vi "DS345 FREQUENCY.vi"(0 "GPIB address":string="19", 1 "amplitude (0 Vrms:0)":cluster{ext, i32} {"?" items=["Vrms", "Vpp", "dBm"]; "?" format="%.3f"}, 2 "output function (sine:0)":u16(ring) items=["sine", "square", "triangle", "ramp", "noise", "arbitrary"], 3 "FREQ. units (Hz:0)":i32(ring) items=["Hz", "KHz.", "MHz."], 4 "frequency":ext format="%.6f", 5 "error in":errorcluster, 6 "phase":ext format="%.3f", 7 "DC offset":ext format="%.3f") -> (8 "error out":errorcluster)   [LabVIEW 2010]
doc: "This subVI specifies the output function, frequency , amplitude,amplitude units and phase of the DS345\nWhen the output function is set to ARBITRARY or NOISE , the frequency or phase may not be changed . \nThe frequency units are used to determine if the frequency quantity needs to be scaled up before sending it to the instrument . \nThe amplitude units can be Vpp, Vrms or dBm ."
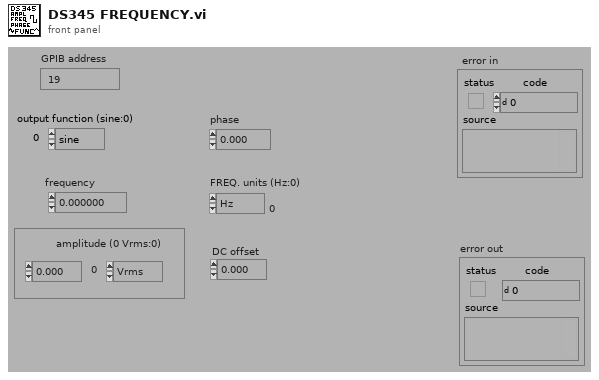
[diagram p1: front panel]
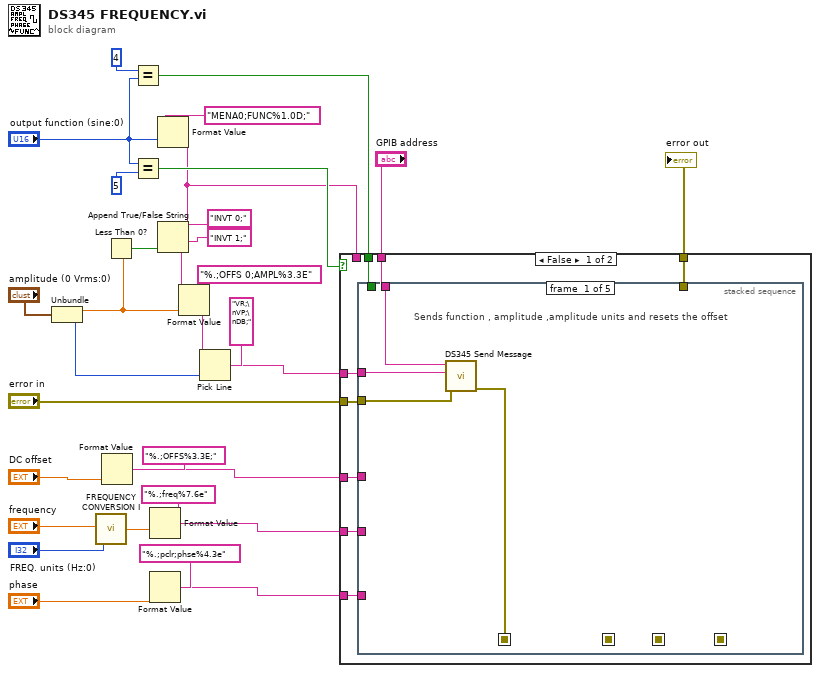
[diagram p0: block diagram]
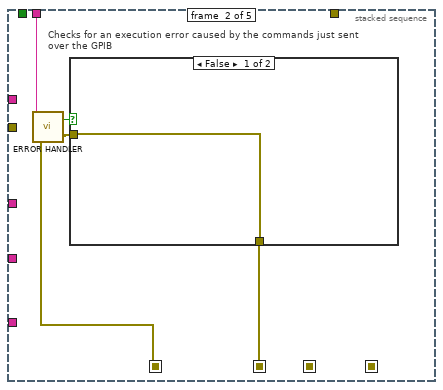
[diagram p2: hidden frame]
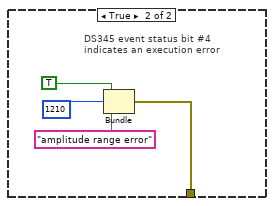
[diagram p3: hidden frame]
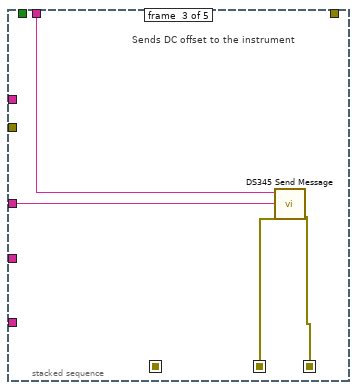
[diagram p4: hidden frame]
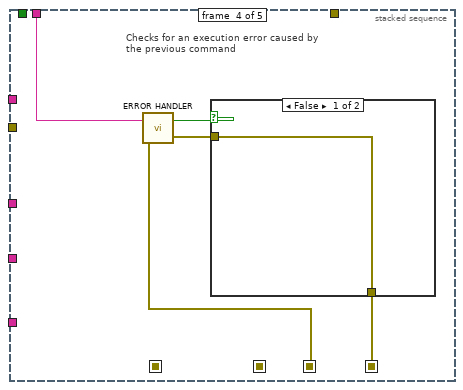
[diagram p5: hidden frame]
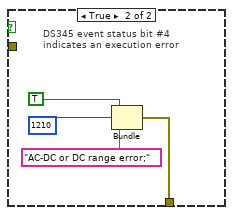
[diagram p6: hidden frame]
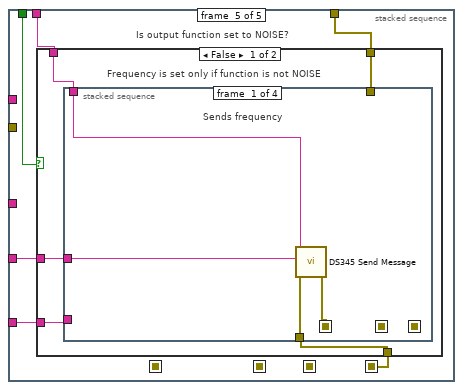
[diagram p7: hidden frame]
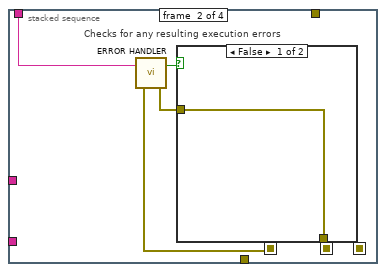
[diagram p8: hidden frame]
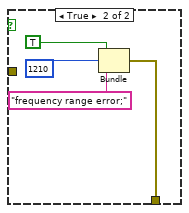
[diagram p9: hidden frame]
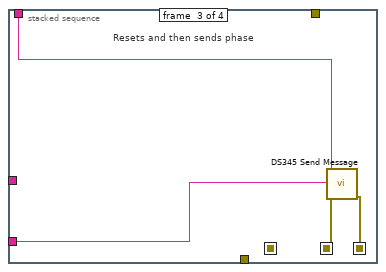
[diagram p10: hidden frame]
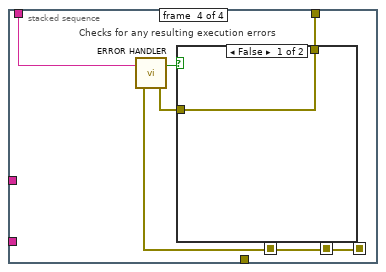
[diagram p11: hidden frame]
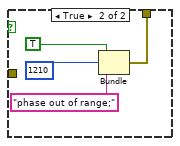
[diagram p12: hidden frame]
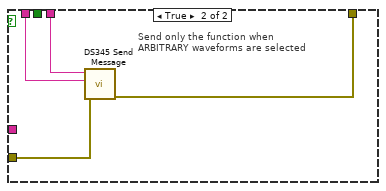
[diagram p14: hidden frame]
diagram:
  n1 = Unbundle("amplitude (0 Vrms:0)") -> (w2:ext, w22:i32)
  n2 = call "FREQUENCY CONVERSION I.vi"("unit"="FREQ. units (Hz:0)", "quantity"="frequency") -> ("output quantity"=w12:ext)
  n3 = Format Value(format string="%.;OFFS%3.3E;", value (0)="DC offset") -> (output string=w15:string)  [unwired: 1 out]
  n4 = Less Than 0?(x=w2) -> (x < 0?=w6:bool)
  n5 = Equal?(x=4, y="output function (sine:0)") -> (x = y?=w19:bool)
  n6 = Equal?(x="output function (sine:0)", y=5) -> (x = y?=w20:bool)
  n7 = Format Value(format string="%.;freq%7.6e", value (0)=w12) -> (output string=w8:string)  [unwired: 1 out]
  n8 = Format Value(format string="%.;pclr;phse%4.3e", value (0)="phase") -> (output string=w9:string)  [unwired: 1 out]
  n9 = Format Value(format string="MENA0;FUNC%1.0D;", value (0)="output function (sine:0)") -> (output string=w3:string)  [unwired: 1 out]
  n10 = Append True/False String(1:w6, 2:"INVT 1;", 3:"INVT 0;", 4:w3) -> (0:w1:string)
  n11 = Format Value(string ("")=w1, format string="%.;OFFS 0;AMPL%3.3E", value (0)=w2) -> (output string=w30:string)
  n12 = Pick Line(string ("")=w30, multi-line string="VR;\nVP;\nDB;", line index=w22) -> (output string=w17:string)
  n13 = case shown="False" w20 {
    tunnel: w19 -> [w40 _]
    tunnel: "GPIB address" -> [w39 w112]
    tunnel: w17 -> [w38 _]
    tunnel: "error in" -> [w37 w110]
    tunnel: w15 -> [w36 _]
    tunnel: [w35 w109] -> w14
    tunnel: w3 -> [_ w111]
    tunnel: w8 -> [w34 _]
    tunnel: w9 -> [w33 _]
    frame False {
      n14 = stacked-sequence {
        seq-local: [w42 _ _ _ _] -> [_ w45 _ _ _]
        seq-local: [_ w46 _ _ _] -> [_ _ w56 _ _]
        seq-local: [_ _ w55 _ _] -> [_ _ _ w61 _]
        seq-local: [_ _ _ w59 _] -> [_ _ _ _ w72]
        tunnel: w39 -> [w44 w49 w58 w63 w74]
        tunnel: w38 -> [w43 _ _ _ _]
        tunnel: w37 -> [w41 _ _ _ _]
        tunnel: w36 -> [_ _ w57 _ _]
        tunnel: [_ _ _ _ w73] -> w35
        tunnel: w40 -> [_ _ _ _ w71]
        tunnel: w34 -> [_ _ _ _ w70]
        tunnel: w33 -> [_ _ _ _ w69]
        frame #0 {
          # "Sends function , amplitude ,amplitude units and resets the offset"
          n15 = call "DS345 Send Message.vi"("address string"=w44, "write buffer"=w43, "error in"=w41) -> ("error out"=w42:errorcluster)  [unwired: 3 in, 3 out]
        }
        frame #1 {
          # "Checks for an execution error caused by the commands just sent \nover the GPIB"
          n16 = call "ERROR HANDLER.vi"("error in"=w45, "GPIB address"=w49) -> ("error out"=w47:errorcluster, "error found"=w48:bool)
          n17 = case shown="False" w48 {
            tunnel: w47 -> [w50 _]
            tunnel: [w50 w51] -> w46
            frame False {
            }
            frame True {
              # "DS345 event status bit #4\nindicates an execution error"
              n18 = Bundle(TRUE, 1210, "amplitude range error") -> (w51:errorcluster)  [unwired: 1 out]
            }
          }
        }
        frame #2 {
          # "Sends DC offset to the instrument"
          n19 = call "DS345 Send Message.vi"("address string"=w58, "write buffer"=w57, "error in"=w56) -> ("error out"=w55:errorcluster)  [unwired: 3 in, 3 out]
        }
        frame #3 {
          # "Checks for an execution error caused by\nthe previous command"
          n20 = call "ERROR HANDLER.vi"("error in"=w61, "GPIB address"=w63) -> ("error out"=w60:errorcluster, "error found"=w62:bool)
          n21 = case shown="False" w62 {
            tunnel: w60 -> [w64 _]
            tunnel: [w64 w65] -> w59
            frame False {
            }
            frame True {
              # "DS345 event status bit #4\nindicates an execution error"
              n22 = Bundle(TRUE, 1210, "AC-DC or DC range error;") -> (w65:errorcluster)  [unwired: 1 out]
            }
          }
        }
        frame #4 {
          # "Is output function set to NOISE?"
          n23 = case shown="False" w71 {
            tunnel: w74 -> [w79 _]
            tunnel: w72 -> [w78 w108]
            tunnel: [w75 w108] -> w73
            tunnel: w70 -> [w77 _]
            tunnel: w69 -> [w76 _]
            frame False {
              # "Frequency is set only if function is not NOISE"
              n24 = stacked-sequence {
                seq-local: [w83 _ _ _] -> [_ w85 _ _]
                seq-local: [_ w84 _ _] -> [_ _ w96 _]
                seq-local: [_ _ w95 _] -> [_ _ _ w100]
                tunnel: w79 -> [w81 w86 w97 w101]
                tunnel: w78 -> [w82 _ _ _]
                tunnel: [_ _ _ w98] -> w75
                tunnel: w77 -> [w80 _ _ _]
                tunnel: w76 -> [_ _ w94 _]
                frame #0 {
                  # "Sends frequency"
                  n25 = call "DS345 Send Message.vi"("address string"=w81, "write buffer"=w80, "error in"=w82) -> ("error out"=w83:errorcluster)  [unwired: 3 in, 3 out]
                }
                frame #1 {
                  # "Checks for any resulting execution errors"
                  n26 = call "ERROR HANDLER.vi"("error in"=w85, "GPIB address"=w86) -> ("error out"=w87:errorcluster, "error found"=w88:bool)
                  n27 = case shown="False" w88 {
                    tunnel: w87 -> [w89 _]
                    tunnel: [w89 w90] -> w84
                    frame False {
                    }
                    frame True {
                      n28 = Bundle(TRUE, 1210, "frequency range error;") -> (w90:errorcluster)  [unwired: 1 out]
                    }
                  }
                }
                frame #2 {
                  # "Resets and then sends phase"
                  n29 = call "DS345 Send Message.vi"("address string"=w97, "write buffer"=w94, "error in"=w96) -> ("error out"=w95:errorcluster)  [unwired: 3 in, 3 out]
                }
                frame #3 {
                  # "Checks for any resulting execution errors"
                  n30 = call "ERROR HANDLER.vi"("error in"=w100, "GPIB address"=w101) -> ("error out"=w99:errorcluster, "error found"=w102:bool)
                  n31 = case shown="False" w102 {
                    tunnel: w99 -> [w103 _]
                    tunnel: [w103 w104] -> w98
                    frame False {
                    }
                    frame True {
                      n32 = Bundle(TRUE, 1210, "phase out of range;") -> (w104:errorcluster)  [unwired: 1 out]
                    }
                  }
                }
              }
            }
            frame True {
            }
          }
        }
      }
    }
    frame True {
      # "Send only the function when \nARBITRARY waveforms are selected"
      n33 = call "DS345 Send Message.vi"("address string"=w112, "write buffer"=w111, "error in"=w110) -> ("error out"=w109:errorcluster)  [unwired: 3 in, 3 out]
    }
  }
  "error out" <- w14
